vi "Refresh UI.vi"(9 "Queue Size ref":refnum<vi>, 10 "Scans Per Write ref":refnum<vi>, 11 "References":T1) -> (0 "error out":errorcluster)   [LabVIEW 2015, in "TDMS datalogger editor node.lvclass"]
uses:
  TDMS datalogger editor node.lvclass
  <vilib>/NI/DCAF/Tag Editor Core/Table API/Table Manager/object ref.ctl
  <vilib>/NI/DCAF/Tag Editor Core/Configuration Editor/Classes/Engine Parent/Engine Parent Editor Node.lvclass
  <vilib>/NI/DCAF/Tag Editor Core/Configuration Editor/Classes/Module editor node/module editor node.lvclass
  TDMS datalogger editor node.lvclass/TDMS datalogger editor node.ctl
  module/configuration/TDMS datalogger configuration.lvclass/TDMS datalogger configuration.ctl
  module/configuration/Read scans per write.vi
  module/configuration/Read queue size.vi
  module/configuration/TDMS datalogger configuration.lvclass
  <vilib>/NI/DCAF/Tag Editor Core/Table API/Table Manager/Table Manager.lvclass
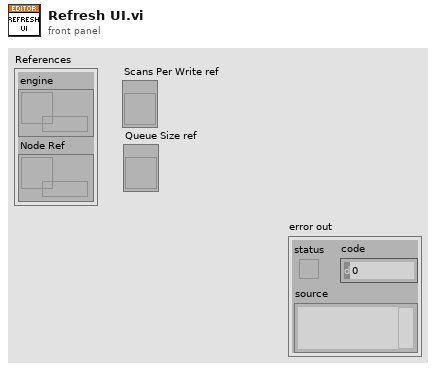
[diagram p1: front panel]
types:
  T1 = typedef "Table Manager.lvlib/Table Manager.lvclass/object ref.ctl" = cluster{"engine":refnum<data-value>, "Node Ref":refnum<data-value>}
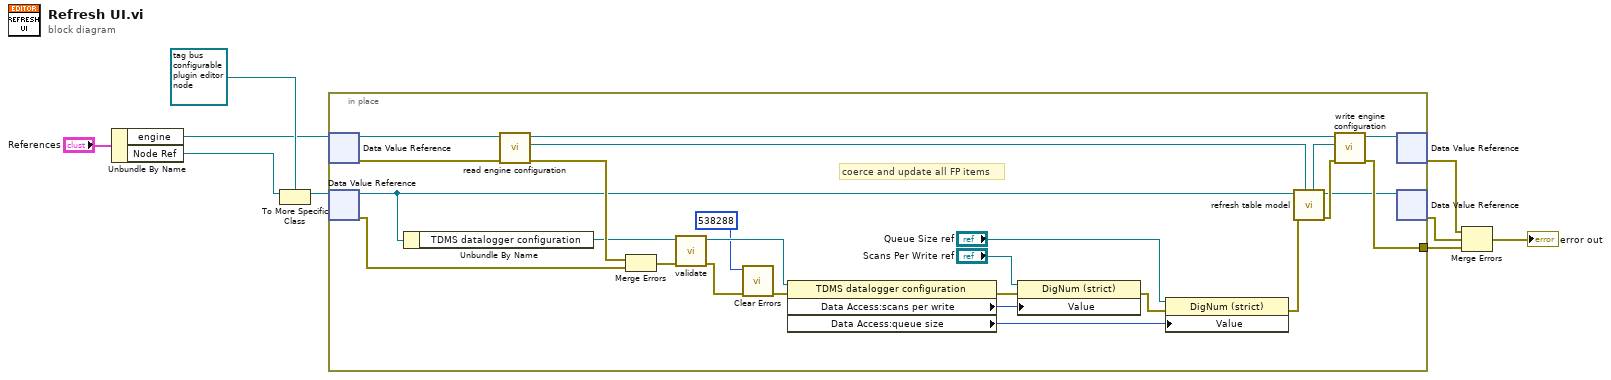
[diagram p0: block diagram]
diagram:
  n1 = Unbundle By Name("References") -> ("engine"=w1:refnum<data-value>, "Node Ref"=w5:refnum<data-value>)
  n2 = To More Specific Class(target class=refnum<data-value> refnum ("data value reference"), reference=w5) -> (specific class reference=w3:refnum<data-value>)  [unwired: 1 in, 1 out]
  n3 = in-place {
    in-place-border: [w18] -> w8
    # "coerce and update all FP items"
    n4 = in-place-dvr #1(w1) -> (w20:refnum<class "Engine Parent Editor Node.lvclass">, w16:errorcluster)
    n5 = in-place-dvr #2(w3) -> (w12:refnum<class "TDMS datalogger editor node.lvclass">, w10:errorcluster)
    n6 = Unbundle By Name(w12) -> ("TDMS datalogger configuration"=w11:refnum<class "TDMS datalogger configuration.lvclass">)
    n7 = call <vilib>:"read engine configuration.vi"("error in"=w16, "Engine Parent Editor Node in"=w20) -> ("error out"=w31:errorcluster, "engine configuration"=w32:refnum<class "engine configuration.lvclass">, "Engine Parent Editor Node out"=w33:refnum<class "Engine Parent Editor Node.lvclass">)  [unwired: 7 in]
    n8 = Merge Errors(w31, w10) -> (w30:errorcluster)
    n9 = call-dynamic "validate.vi"("error in"=w30, "TDMS datalogger configuration in"=w11) -> ("error out"=w22:errorcluster, "TDMS datalogger configuration out"=w29:refnum<class "TDMS datalogger configuration.lvclass">)  [unwired: 8 in]
    n10 = call <vilib>:"Clear Errors.vi"("error in (no error)"=w22, "specific error code to clear (0: all)"=538288) -> ("error out"=w23:errorcluster)  [unwired: 4 in, 1 out]
    n11 = property class="TDMS datalogger configuration"(reference=w29, error in=w23) -> (error out=w26:errorcluster, "Data Access:scans per write"=w28:u16, "Data Access:queue size"=w27:u16)  [unwired: 1 out]
    n12 = property on="Property Node" class="DigNum (strict)"(reference="Scans Per Write ref", error in=w26, "Value"=w28) -> (error out=w25:errorcluster)  [unwired: 1 out]
    n13 = property on="Property Node" class="DigNum (strict)"(reference="Queue Size ref", error in=w25, "Value"=w27) -> (error out=w24:errorcluster)  [unwired: 1 out]
    n14 = call "refresh table model.vi"("engine configuration"=w32, "error in"=w24, "TDMS editor node"=w12) -> ("error out"=w17:errorcluster, "TDMS editor node out"=w15:refnum<class "TDMS datalogger editor node.lvclass">, "engine configuration out"=w34:refnum<class "engine configuration.lvclass">)  [unwired: 6 in]
    n15 = call <vilib>:"write engine configuration.vi"("error in"=w17, "engine configuration"=w34, "Engine Parent Editor Node in"=w33) -> ("error out"=w18:errorcluster, "Engine Parent Editor Node out"=w19:refnum<class "Engine Parent Editor Node.lvclass">)  [unwired: 7 in]
    n16 = in-place-dvr #1(w19) -> (w6:errorcluster)  [unwired: 1 out]
    n17 = in-place-dvr #2(w15) -> (w2:errorcluster)  [unwired: 1 out]
  }
  n18 = Merge Errors(w6, w2, w8) -> (→"error out":errorcluster)
